vi "HOST_timesharing+input.vi"() -> ()   [LabVIEW 2020]
uses:
  <vilib>/userDefined/Silver/nirio_resource_slv.ctl
  Controls/Clock Select.ctl
  <vilib>/FPGAPlugInAG/PXIe-7972R/niLvFpga_Open_PXIe-7972R.vi
  <vilib>/rvi/interface/common/dynamic/niFpgaDynamicAddResources.vi
  <vilib>/rvi/interface/common/niFpgaWaitOnOcc.vi
  <vilib>/Utility/error.llb/Error Cluster From Error Code.vi
  <vilib>/rvi/errors/niLvFpgaAdjustHostInterfaceError.vi
  <instrlib>/_niInstr/Streaming/v1/Host/Public/Start Finite Stream.vi
  <instrlib>/_niInstr/Streaming/v1/Host/Public/Wait for Stream.vi
  <instrlib>/_niInstr/Streaming/v1/Host/Public/Start Continuous Stream.vi
  <vilib>/FPGAPlugInAG/Dynamic/niLvFpga_Close_Dynamic.vi
  <vilib>/rvi/interface/nirviOpenFPGA/nirviOpenFPGA.xnode
  FPGA Bitfiles/rfsignal_FPGATarget_timecycling+PID_CIi3kE6w0Lk.lvbitx
  <vilib>/rvi/interface/nirviMethod/nirviMethod.xnode
  <vilib>/rvi/interface/nirviReadWriteControl/nirviReadWriteControl.xnode
  <vilib>/rvi/interface/nirviCloseFPGA/nirviCloseFPGA.xnode
  <vilib>/rvi/errors/niLvFpgaMergeErrorWithErrorCode.vi
  <instrlib>/_niInstr/Streaming/v1/Host/niInstr Streaming v1 Host.lvlib
  <vilib>/rvi/interface/Simulation/niFpgaSimulationCallBeginRW.vi
  <vilib>/FPGAPlugInAG/Dynamic/niLvFpga_ConfigureFifo_Dynamic.vi
  <vilib>/FPGAPlugInAG/Dynamic/niLvFpga_StartFifo_Dynamic.vi
  NiFpgaLv.dll
  <vilib>/FPGAPlugInAG/Dynamic/niLvFpga_WriteFifo_Dynamic.vi
panel:
  in  "Input pass through\nmode":enum16{"Wire", "Accum", "Accum-edge"}(ring)
  in  "Ch 1 # of waves":i8=2
  in  "Ch 0 # of waves":i8=2
  in  "Wave Reader CH 1":fxp<+/-,64,32>[](array[numeric])=[27300000.0, 28000000.0, 28000000.0, 32000000.0, 21000000.0, 25000000.0, 30000000.0, 34000000.0] format="%_6p"
  in  "Gain CH 1 (multiplicative)":fxp<+,32,4>[](array[numeric])=[0.8500000014901161, 1.3999999985098839, 0.9999999925494194, 1.300000000745058, 1.0, 1.0, 1.0, 1.0]
  in  "Clean 2x edge cycles":i32=5
  in  "Time per beam in us":i32=10
  in  "stop":bool
  in  "Gain CH 0 (multiplicative)":fxp<+,32,4>[](array[numeric])=[0.9999999962747097, 0.6999999992549419, 1.199999999254942, 0.5, 1.0, 1.0, 1.0, 1.0]
  in  "Wave Reader CH 0":fxp<+/-,64,32>[](array[numeric])=[22000000.0, 24000000.0, 28000000.0, 32000000.0, 21000000.0, 25000000.0, 30000000.0, 34000000.0] format="%_6p"
  out "AO":waveform(dbl)(graph)={"t0"=timestamp(0.0056 s since 1904-01-01), "dt"=1.220703125e-08, "Y"=array[65536 elements]}
  in  "Magnitude Initialization\nVpp":dbl[](array[numeric])=[0.1, 0.1] format="%0.2p"
  in  "Frequencies (Hz)":dbl[](array[numeric])=[10000.0, 10000.0] format="%5.0p"
  in  "Signal Type":T1(ring)
  in  "Sampling Info":cluster{"Fs":dbl, "#s":dbl}={"Fs"=163840000.0, "#s"=65536.0} {"Fs" format="%#_5p"}
  out "Error Out":errorcluster
  in  "Update Waveform":bool
  in  "AO Channel":T2(ring)
  in  "Clock Select":T3 items=["Internal Clock", "Internal Clock w/ Ref via CLK/REF IN", "Internal Clock w/ Ref via Sync Clock", "External Clock via CLK/REF IN"]
  in  "Rate of External Sample Clock (MHz)":u16=100 min=60 max=100 step=1
  in  "RIO Resource":T4="PXI1Slot5"
  # "Analog In"
  # "Waveform Initialization"
  # "Ch 1 Output Waveforms"
  # "Ch 0 Output Waveforms"
  # "DO NOT CHANGE"
  # "Ch0"
  # "Ch1"
  # "Don't change"
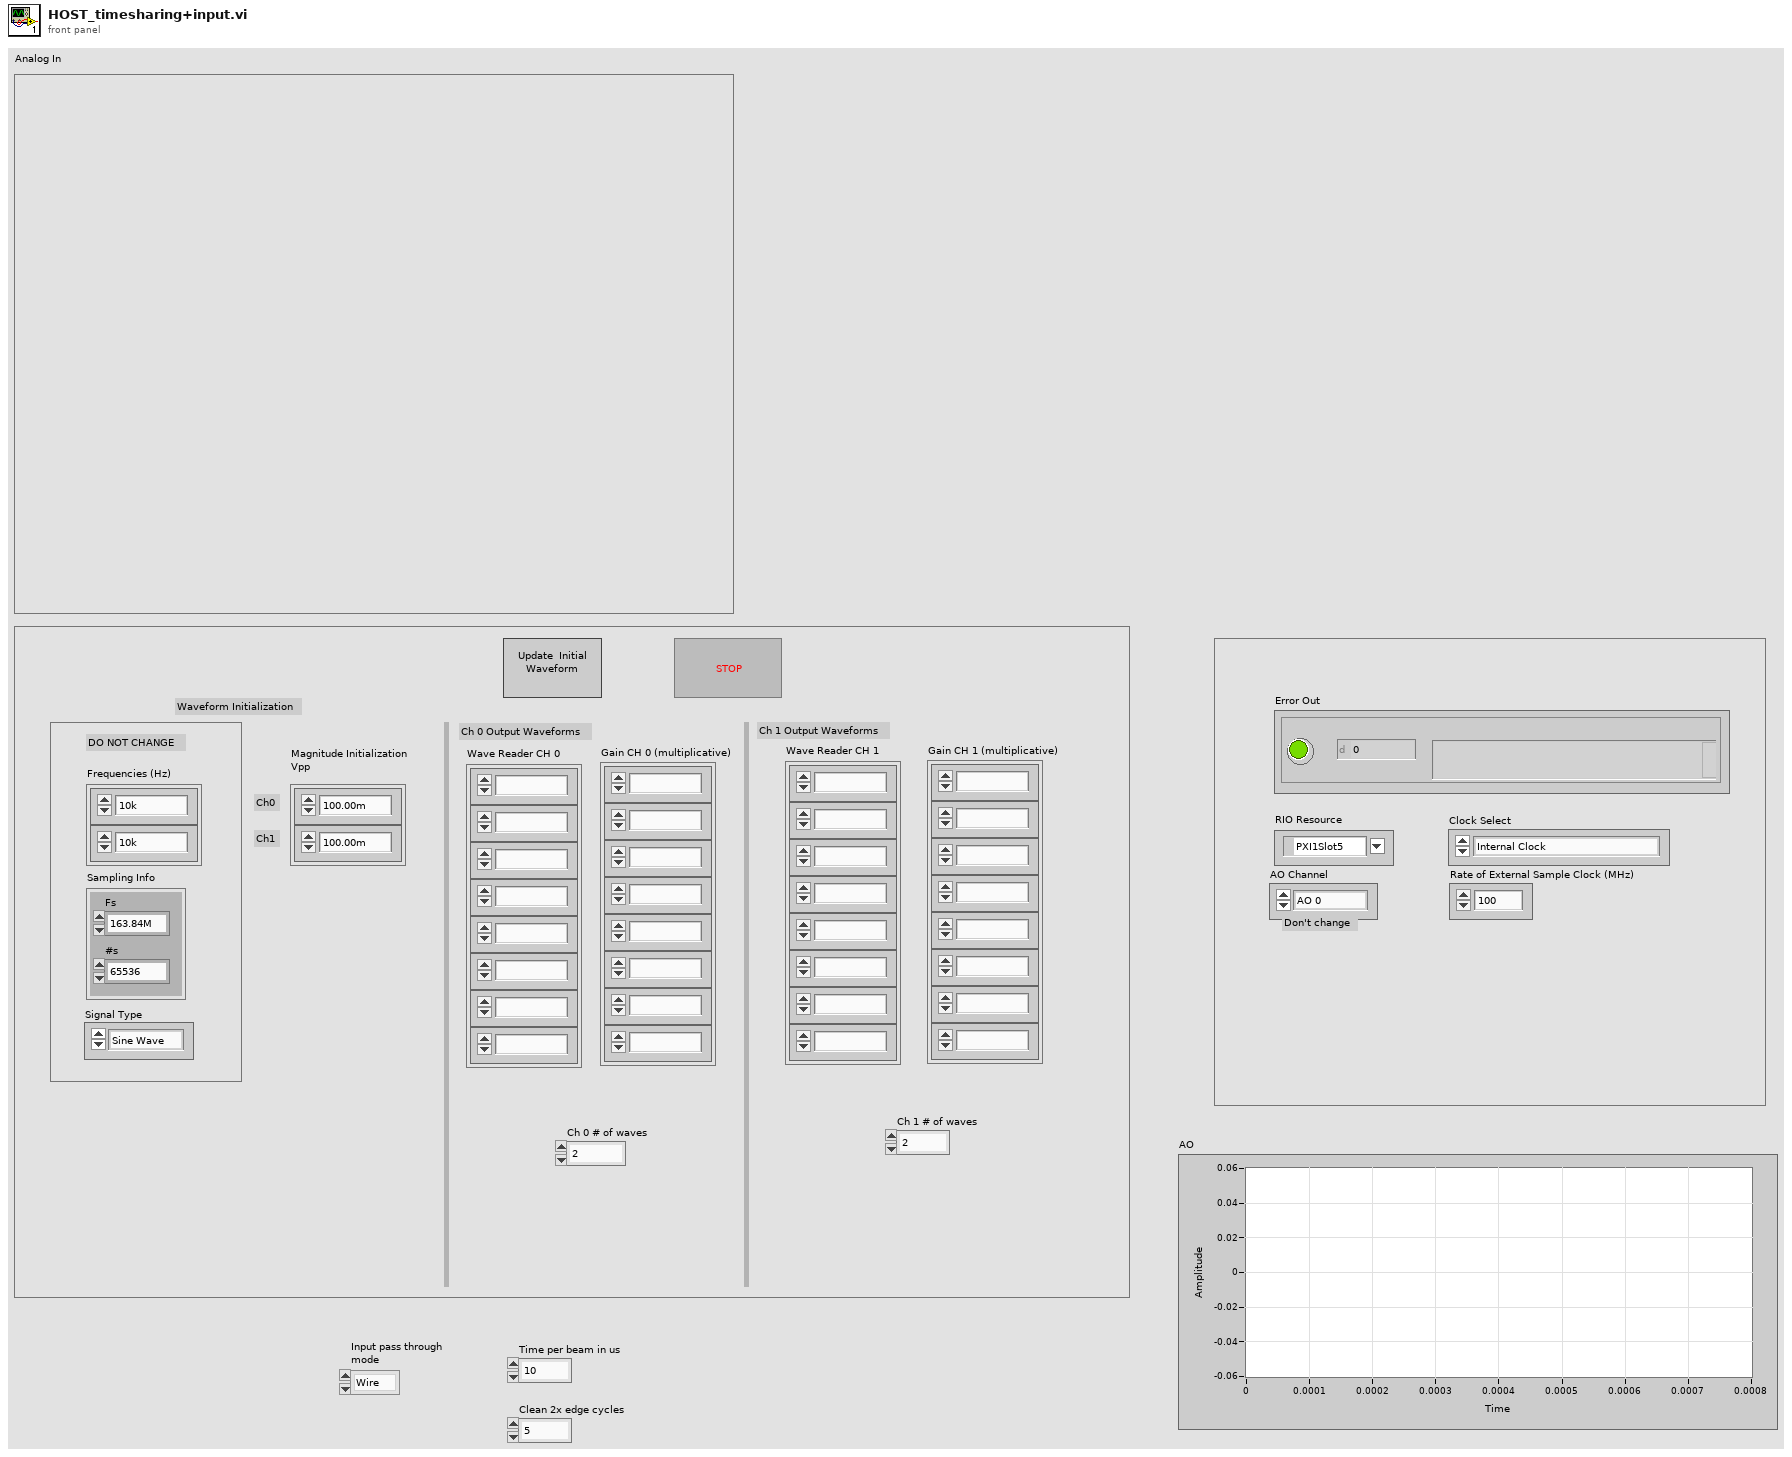
[diagram p1: front panel]
types:
  T1 = enum16{"Sine Wave", "Triangle Wave", "Square Wave", "Sawtooth Wave"}
  T2 = enum8{"AO 0", "AO 1", "AO 2", "AO 3", "AO 0, AO 1, AO 2, AO 3", "None"}
  T3 = typedef "Clock Select.ctl" = u16
  T4 = typedef "nirio_resource_slv.ctl" = tag
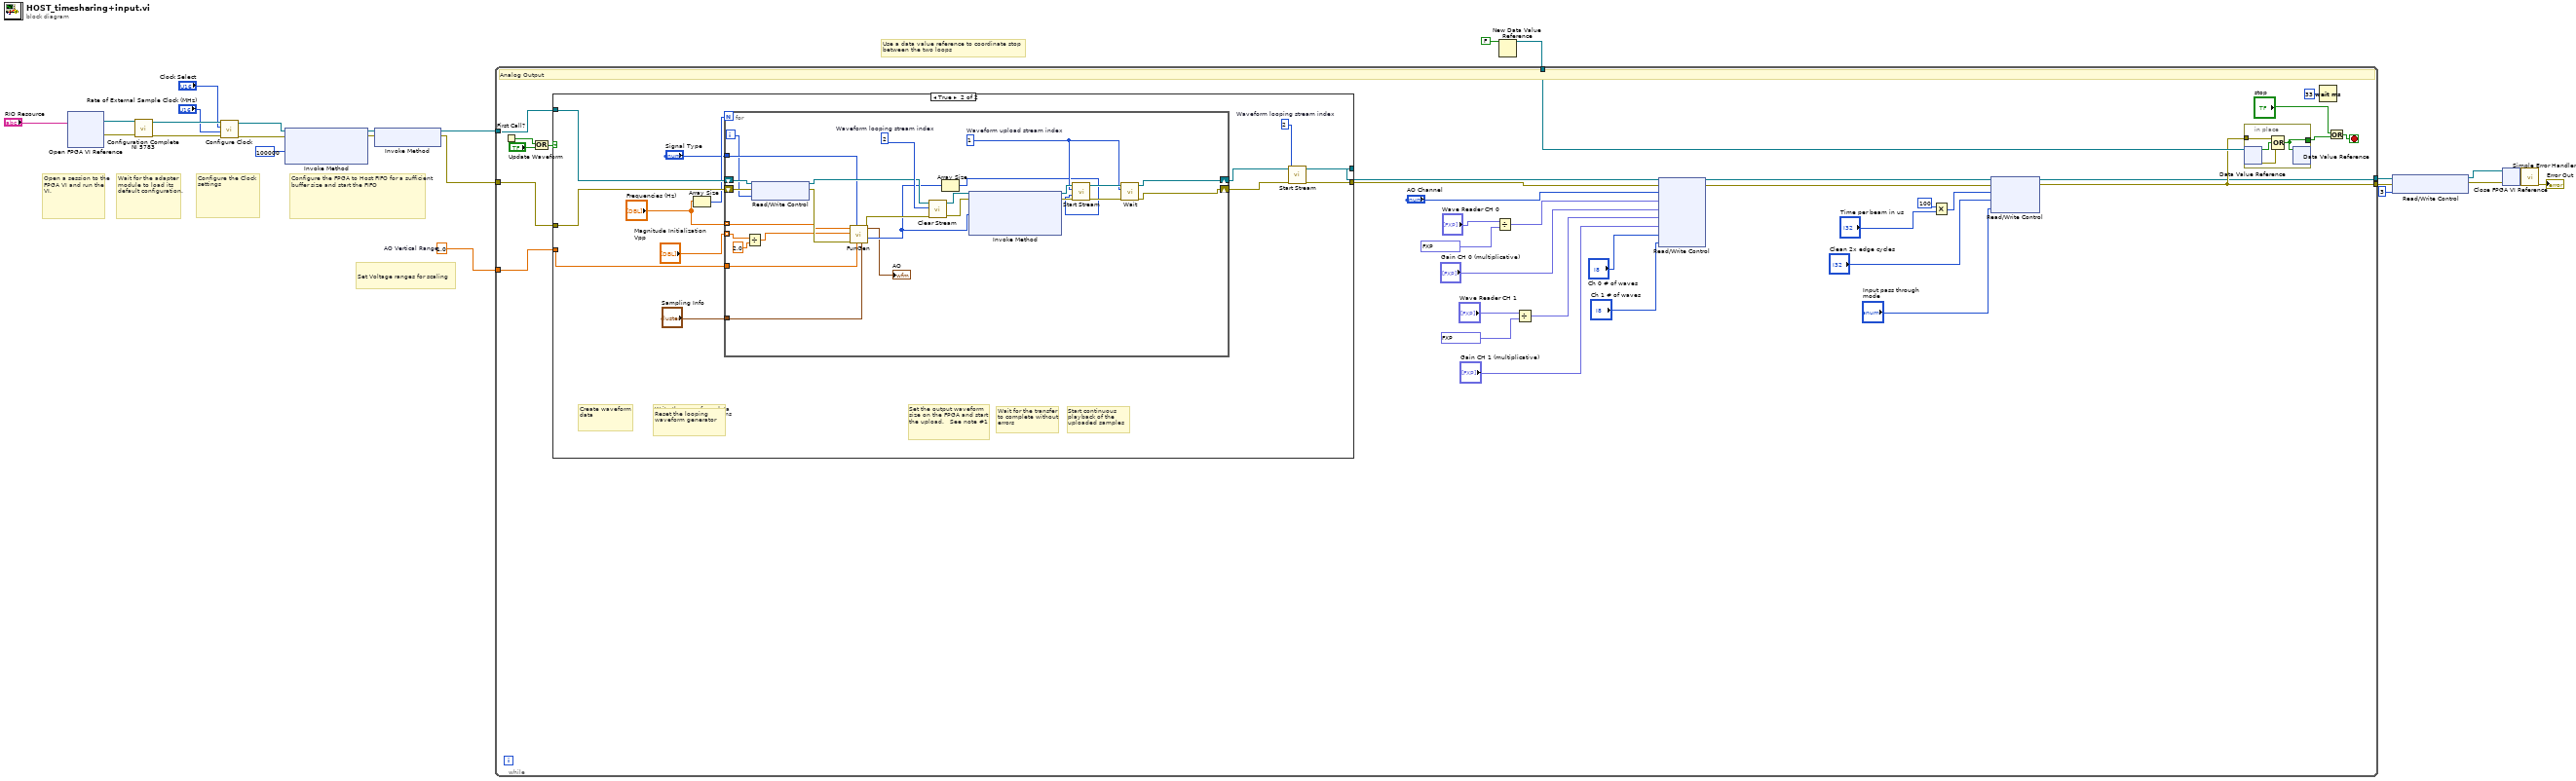
[diagram p0: block diagram]
diagram:
  w12 = 1.0  # AO Vertical Range
  # "Use a data value reference to coordinate stop between the two loops"
  # "Set Voltage ranges for scaling"
  # "Configure the Clock settings"
  # "Configure the FPGA to Host FIFO for a sufficient buffer size and start the FIFO"
  # "Wait for the adapter module to load its default configuration."
  # "Open a session to the FPGA VI and run the VI."
  n1 = xnode "Open FPGA VI Reference"("resource name"="RIO Resource") -> ("FPGA VI Reference Out"=w10:refnum<k20>, "error out"=w9:errorcluster)  [unwired: 1 in]
  n2 = call "Configuration Complete NI 5783.vi"("error in"=w9, "FPGA VI Reference In"=w10) -> ("error out"=w20:errorcluster, "FPGA VI Reference Out"=w21:refnum<k20>)  [unwired: 7 in, 1 out]
  n3 = call "Configure Clock.vi"("error in (no error)"=w20, "Rate of External Sample Clock (MHz)"="Rate of External Sample Clock (MHz)", "Clock Select"="Clock Select", "FPGA VI Reference In"=w21) -> ("error out"=w18:errorcluster, "FPGA VI Reference Out"=w19:refnum<k20>)  [unwired: 3 in, 3 out]
  n4 = xnode "Invoke Method"("FPGA VI Reference In"=w19, "error in"=w18, "Requested Depth"=u32 100000) -> ("FPGA VI Reference Out"=w24:refnum<k20>, "error out"=w23:errorcluster)  [unwired: 1 out]
  n5 = xnode "Invoke Method"("FPGA VI Reference In"=w24, "error in"=w23) -> ("FPGA VI Reference Out"=w3:refnum<k20>, "error out"=w2:errorcluster)
  n6 = New Data Value Reference(data value=FALSE ("Stopped")) -> (data value reference=w1:refnum<data-value>)  [unwired: 1 in, 1 out]
  n7 = while {
    tunnel: w2 -> [w51]
    tunnel: [w39] -> w8
    tunnel: w3 -> [w57]
    tunnel: [w38] -> w7
    tunnel: w1 -> [w52]
    tunnel: w12 -> [w50]
    stop <- w46 stop-if-true
    # "Analog Output"
    n8 = First Call?() -> (First Call?: T/F=w53:bool)
    n9 = Or(x=w53, y="Update Waveform") -> (x .or. y?=w54:bool)
    n10 = case shown="True" w54 {
      tunnel: [w63 w76] -> w49
      tunnel: [w62 w75] -> w48
      tunnel: w57 -> [w63 w73]
      tunnel: w51 -> [w62 w72]
      tunnel: w50 -> [_ w74]
      frame False {
      }
      frame True {
        w71 = 2  # Waveform looping stream index
        # "Loop over the waveforms to combine"
        # "Reset the looping waveform generator"
        # "Start continuous playback of the uploaded samples"
        # "Wait for the transfer to complete without errors"
        # "Set the output waveform size on the FPGA and start the upload.   See note #1"
        # "Write the waveform data to the FPGA for generation"
        # "Create waveform data"
        n11 = Array Size(array="Frequencies (Hz)") -> (size(s)=w66:i32)
        n12 = for {
          N: w66 -> [_]
          tunnel: w74 -> [w92]
          shift-right: [w86] -> w70
          shift-left: w73 -> [w91]
          shift-right: [w85] -> w69
          shift-left: w72 -> [w89]
          tunnel: "Frequencies (Hz)" -> [w84] mode=indexing
          tunnel: "Magnitude Initialization\nVpp" -> [w80] mode=indexing
          tunnel: "Sampling Info" -> [w83]
          tunnel: "Signal Type" -> [w82]
          i -> [w81]
          w93 = 2  # Waveform looping stream index
          w98 = 1  # Waveform upload stream index
          n13 = Divide(x=w80, y=2.0) -> (x/y=w79:dbl)
          n14 = xnode "Read/Write Control"("FPGA VI Reference In"=w91, "error in"=w89, "Upload selector"=w81) -> ("FPGA VI Reference Out"=w90:refnum<k20>, "error out"=w88:errorcluster)
          n15 = call "FunGen.vi"("sampling info"=w83, "range (Vpp)"=w92, "signal type"=w82, "error in (no error)"=w88, "amplitude"=w79, "frequency"=w84) -> ("error out"=w94:errorcluster, "Waveform Data"=w87:i16[], "Output Waveform (V)"=→"AO":waveform(dbl))  [unwired: 2 in, 1 out]
          n16 = call <instrlib>:"Clear Stream.vi"("error in (no error)"=w94, "stream index"=w93, "refnum in"=w90) -> ("error out"=w96:errorcluster, "refnum out"=w97:refnum<k20>)  [unwired: 7 in]
          n17 = Array Size(array=w87) -> (size(s)=w95:i32)
          n18 = xnode "Invoke Method"("FPGA VI Reference In"=w97, "error in"=w96, "Data"=w87) -> ("FPGA VI Reference Out"=w102:refnum<k20>, "error out"=w101:errorcluster)  [unwired: 1 in, 1 out]
          n19 = call-poly <instrlib>:"Start Stream.vi"("error in (no error)"=w101, "num samples"=w95, "stream index"=w98, "refnum in"=w102) -> ("error out"=w99:errorcluster, "refnum out"=w100:refnum<k20>)  [unwired: 6 in]
          n20 = call-poly <instrlib>:"Wait.vi"("error in (no error)"=w99, "stream index"=w98, "refnum in"=w100) -> ("error out"=w85:errorcluster, "refnum out"=w86:refnum<k20>)  [unwired: 5 in, 2 out]
        }
        n21 = call-poly <instrlib>:"Start Stream.vi"("error in (no error)"=w69, "stream index"=w71, "refnum in"=w70) -> ("error out"=w75:errorcluster, "refnum out"=w76:refnum<k20>)  [unwired: 7 in]
      }
    }
    n22 = Divide(x="Wave Reader CH 0", y=fxp<+,32,16> 6103.515625) -> (x/y=w33:fxp<+,32,16>[])
    n23 = Divide(x="Wave Reader CH 1", y=fxp<+,32,16> 6103.515625) -> (x/y=w30:fxp<+,32,16>[])
    n24 = xnode "Read/Write Control"("FPGA VI Reference In"=w49, "error in"=w48, "AO Channel"="AO Channel", "Wave 1"=w33, "Amp 1"="Gain CH 0 (multiplicative)", "Wave 2"=w30, "Amp 2"="Gain CH 1 (multiplicative)", "Ch 0 size"="Ch 0 # of waves", "Ch 1 size"="Ch 1 # of waves") -> ("FPGA VI Reference Out"=w41:refnum<k20>, "error out"=w40:errorcluster)
    n25 = Multiply(x=100, y="Time per beam in us") -> (x*y=w35:i32)
    n26 = xnode "Read/Write Control"("FPGA VI Reference In"=w41, "error in"=w40, "Timeshare"=w35, "Edge size"="Clean 2x edge cycles", "Pass selector"="Input pass through\nmode") -> ("FPGA VI Reference Out"=w38:refnum<k20>, "error out"=w39:errorcluster)
    n27 = in-place {
      in-place-border: [w59] -> w45
      in-place-border: w39 -> [w61]
      n28 = in-place-dvr #1(w52) -> (w60:bool, w58:errorcluster)
      n29 = Compound Arithmetic op=OR(w61, w60, w58) -> (w59:bool)
      n30 = in-place-dvr #1(w59) -> ()  [unwired: 2 out]
    }
    n31 = Wait (ms)(milliseconds to wait=u32 33) -> ()  [unwired: 1 out]
    n32 = Or(x="stop", y=w45) -> (x .or. y?=w46:bool)
  }
  n33 = xnode "Read/Write Control"("FPGA VI Reference In"=w7, "error in"=w8, "stream.request state 2"=3) -> ("FPGA VI Reference Out"=w4:refnum<k20>, "error out"=w6:errorcluster)
  n34 = xnode "Close FPGA VI Reference"("FPGA VI Reference In"=w4, "error in"=w6) -> ("error out"=w15:errorcluster)
  n35 = call <vilib>:"Simple Error Handler.vi"("error in (no error)"=w15) -> ("error out"=→"Error Out":errorcluster)  [unwired: 4 in, 4 out]
